vi "ExecuteSetSaveChangesAutoSelection.vi"(8 "error in (no error)":errorcluster, 11 "New SaveChangesAutoSelection value":i32) -> (0 "error out":errorcluster, 3 "Previous SaveChangesAutoSelection value":i32)   [LabVIEW 2014]
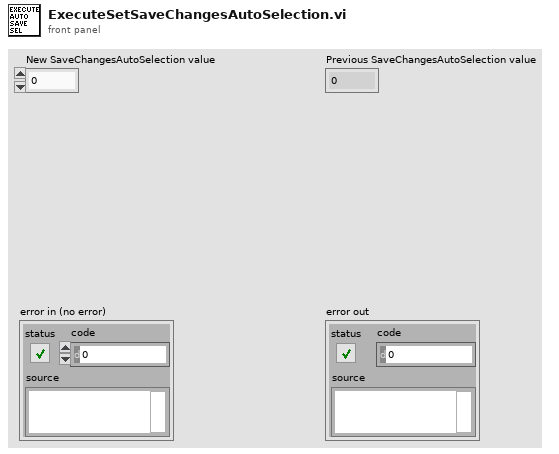
[diagram p1: front panel]
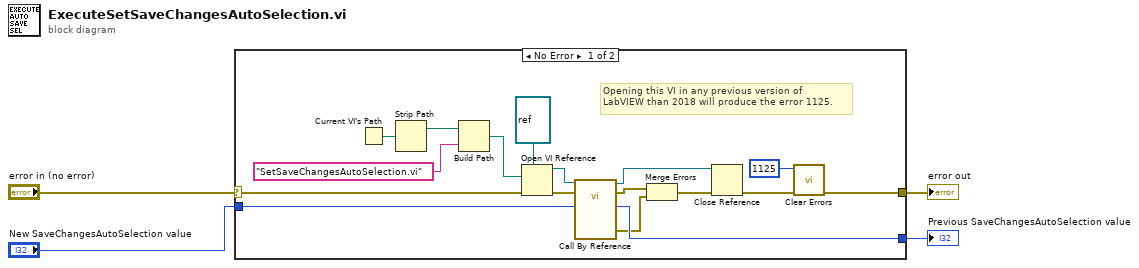
[diagram p0: block diagram]
diagram:
  n1 = case shown="No Error" "error in (no error)" {
    selector: "error in (no error)" -> [w5 w22]
    tunnel: [w11 w22] -> w3
    tunnel: "New SaveChangesAutoSelection value" -> [w9 _]
    tunnel: [w8 _] -> w1
    frame No Error {
      # "Opening this VI in any previous version of\nLabVIEW than 2018 will produce the error 1125."
      n2 = Current VI's Path() -> (path=w19:path)
      n3 = Strip Path(path=w19) -> (stripped path=w20:path)  [unwired: 1 out]
      n4 = Build Path(base path=w20, name or relative path="SetSaveChangesAutoSelection.vi") -> (appended path=w18:path)
      n5 = Open VI Reference(type specifier VI Refnum (for type only)=refnum<vi> refnum, vi path=w18, error in (no error)=w5) -> (vi reference=w16:refnum<vi>, error out=w15:errorcluster)  [unwired: 3 in]
      n6 = call-by-ref "?"(reference=w16, error in=w15, "New SaveChangesAutoSelection value"=w9) -> (reference out=w13:refnum<vi>, error out=w12:errorcluster, 0:"error out"=w6:errorcluster, "Previous SaveChangesAutoSelection value"=w8:i32)  [unwired: 9 in]
      n7 = Merge Errors(w12, w6) -> (w7:errorcluster)
      n8 = Close Reference(reference=w13, error in (no error)=w7) -> (error out=w14:errorcluster)
      n9 = call <vilib>:"Clear Errors.vi"("error in (no error)"=w14, "specific error code to clear (0: all)"=1125) -> ("error out"=w11:errorcluster)  [unwired: 4 in, 1 out]
    }
    frame Error {
    }
  }
  "error out" <- w3
  "Previous SaveChangesAutoSelection value" <- w1
